vi "McP ScanIndicator.vi"(1 "Grating factor":dbl format="%.2f", 2 "Current Wavelength":dbl=900.0 format="%.2f", 3 "New Wavelength":dbl=500.0 format="%.2f", 4 "MoveTime(ms)":dbl=20.0 format="%.2f") -> ()   [LabVIEW 2019]
uses:
  Globals and TypeDefs/Global Varibal Control.vi
panel:
  out "?":string
  out "Counter Reading":dbl min=0.0
  out "Wavelength (nm)":dbl(knob) caption="Spectrometer Moving" scale=800.0..899.9997799999999
  out "TimeRemaining":dbl min=0.0 format="%.1f"
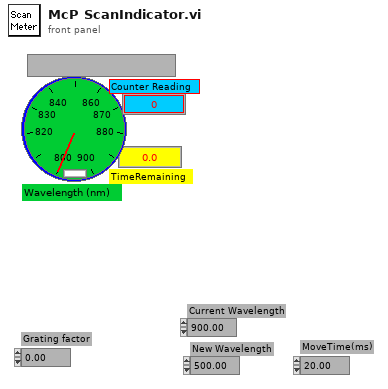
[diagram p1: front panel]
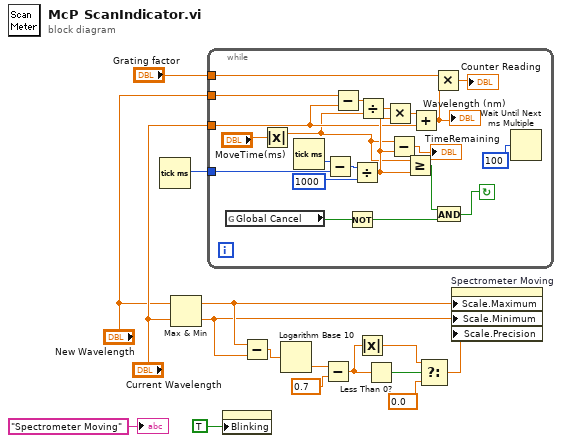
[diagram p0: block diagram]
diagram:
  n1 = Tick Count (ms)() -> (millisecond timer value=w14:u32)
  n2 = Max & Min(x="New Wavelength", y="Current Wavelength") -> (max(x,y)=w10:dbl, min(x,y)=w9:dbl)
  n3 = while {
    tunnel: "Grating factor" -> [w25]
    tunnel: "Current Wavelength" -> [w27]
    tunnel: "New Wavelength" -> [w32]
    tunnel: w14 -> [w36]
    stop <- w17 continue-if-true
    n4 = global read "Global Varibal Control.vi" "Global Cancel"() -> (w19:bool)
    n5 = Absolute Value(x="MoveTime(ms)") -> (abs(x)=w21:dbl)
    n6 = Tick Count (ms)() -> (millisecond timer value=w37:u32)
    n7 = Subtract(x=w37, y=w36) -> (x-y=w35:u32)
    n8 = Subtract(x=w32, y=w27) -> (x-y=w31:dbl)
    n9 = Not(x=w19) -> (.not. x?=w20:bool)
    n10 = Divide(x=w35, y=u32 1000) -> (x/y=w30:dbl)
    n11 = Divide(x=w31, y=w21) -> (x/y=w29:dbl)
    n12 = Multiply(x=w29, y=w30) -> (x*y=w28:dbl)
    n13 = Subtract(x=w21, y=w30) -> (x-y=→"TimeRemaining":dbl)
    n14 = Greater Or Equal?(x=w21, y=w30) -> (x >= y?=w18:bool)
    n15 = Add(x=w28, y=w27) -> (x+y=w24:dbl)
    "Wavelength (nm)" <- w24
    n16 = Multiply(x=w25, y=w24) -> (x*y=→"Counter Reading":dbl)
    n17 = And(x=w18, y=w20) -> (x .and. y?=w17:bool)
    n18 = Wait Until Next ms Multiple(millisecond multiple=u32 100) -> ()  [unwired: 1 out]
  }
  n19 = property class="Str"("Blinking"=TRUE) -> ()  [unwired: 2 in, 2 out]
  n20 = Subtract(x=w10, y=w9) -> (x-y=w6:dbl)
  n21 = Logarithm Base 10(1:w6) -> (0:w8:dbl)
  n22 = Subtract(x=w8, y=0.7) -> (x-y=w4:dbl)
  n23 = Absolute Value(x=w4) -> (abs(x)=w1:dbl)
  n24 = Less Than 0?(x=w4) -> (x < 0?=w5:bool)
  n25 = Select(t=w1, s=w5, f=0.0) -> (s? t:f=w2:dbl)
  n26 = property on="Spectrometer Moving" class="Knob (strict)"("Scale.Maximum"=w10, "Scale.Minimum"=w9, "Scale.Precision"=w2) -> ()  [unwired: 2 in, 2 out]
  "?" <- "Spectrometer Moving"
